vi "newsubvi Robot Get XY.vi"(0 "VISA In":refnum<visa-resource-name>="COM8") -> (1 "VISA Out":refnum<visa-resource-name>, 2 "XPosition":i32, 3 "YPosition":i32, 4 "error out":errorcluster)   [LabVIEW 2012]
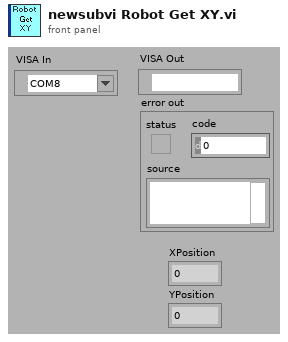
[diagram p1: front panel]
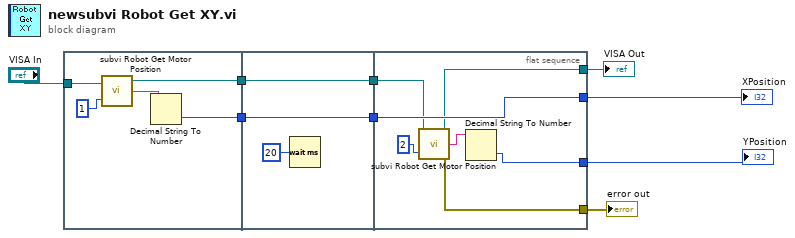
[diagram p0: block diagram]
diagram:
  n1 = flat-sequence {
    tunnel: [w12] -> w8
    tunnel: "VISA In" -> [w11]
    tunnel: [w10] -> w3
    tunnel: [w16] -> w5
    tunnel: w8 -> [w16]
    tunnel: [w15] -> w4
    tunnel: w3 -> [w15]
    tunnel: [w22] -> w9
    tunnel: w5 -> [w22]
    tunnel: [w21] -> w7
    tunnel: w4 -> [w20]
    tunnel: [w19] -> w2
    tunnel: [w18] -> w1
    frame #0 {
      n2 = call "subvi Robot Get Motor Position.vi"("VISA In"=w11, "Motor Number"=1) -> ("VISA Out"=w10:refnum<visa-resource-name>, "Motor Position"=w13:string)  [unwired: 2 out]
      n3 = Decimal String To Number(string=w13) -> (number=w12:i32)  [unwired: 3 out]
    }
    frame #1 {
      n4 = Wait (ms)(milliseconds to wait=u32 20) -> ()  [unwired: 1 out]
    }
    frame #2 {
      n5 = call "subvi Robot Get Motor Position.vi"("VISA In"=w20, "Motor Number"=2) -> ("VISA Out"=w19:refnum<visa-resource-name>, "Motor Position"=w23:string, "error out"=w18:errorcluster)  [unwired: 1 out]
      n6 = Decimal String To Number(string=w23) -> (number=w21:i32)  [unwired: 3 out]
    }
  }
  "XPosition" <- w9
  "YPosition" <- w7
  "VISA Out" <- w2
  "error out" <- w1
